vi "Kinect Example.vi"() -> ()   [LabVIEW 2011]
doc: "This example VI shows off the functionality of the new and improved Kinect API."
uses:
  Kinect Library/Kinect Type Defs/Color Image Format.ctl
  Kinect Library/Kinect Type Defs/Depth Image Format.ctl
  Kinect Library/Kinect Library.lvlib
panel:
  in  "Depth Image Format":T1
  in  "Color Image Format":T2
  in  "Kinect Sensor Index":i32
  out "Kinect Properties":T3(array[cluster])
  out "BeamAngle":dbl
  out "SoundSourceAngleConfidence":dbl
  out "SoundSourceAngle":dbl(slide) scale=-90.0..90.0
  out "Skeletal Data":T4(array[cluster])
  out "Depth Image":T5(plugin-control)
  out "Color Image":T5(plugin-control)
  in  "Stop":bool
  out "error out":errorcluster
  out "Move Success?":bool
  out "Number of Kinects Attached":i32
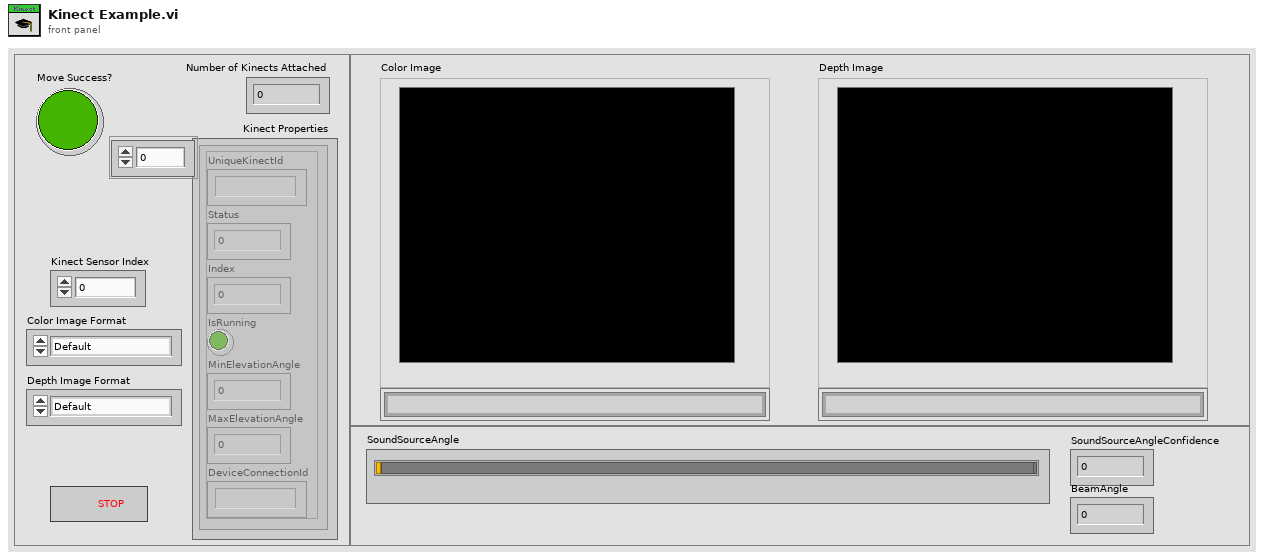
[diagram p1: front panel]
types:
  T1 = typedef "Kinect Library.lvlib/Depth Image Format.ctl" = enum16{"Default", "Undefined", "Resolution640x480Fps30", "Resolution320x240Fps30", "Resolution80x60Fps30"}
  T2 = typedef "Kinect Library.lvlib/Color Image Format.ctl" = enum16{"Default", "Undefined", "RgbResolution640x480Fps30", "RgbResolution1280x960Fps12", "YuvResolution640x480Fps15", "RawYuvResolution640x480Fps15"}
  T3 = cluster{"UniqueKinectId":string, "Status":i32, "Index":i32, "IsRunning":bool, "MinElevationAngle":i32, "MaxElevationAngle":i32, "DeviceConnectionId":string}[]
  T4 = cluster{"ClippedEdges":i32, cluster{"JointType":i32, cluster{"X":sgl, "Y":sgl, "Z":sgl}, "TrackingState":i32}[], cluster{"X":sgl, "Y":sgl, "Z":sgl}, "TrackingId":i32, "TrackingState":i32}[]
  T5 = typedef "IMAQ Image.ctl" = refnum<image>
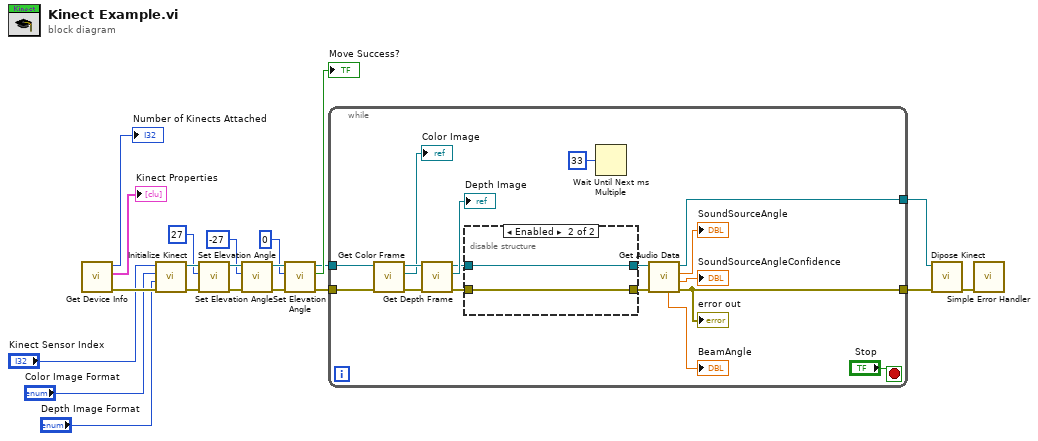
[diagram p0: block diagram]
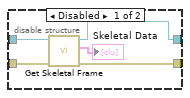
[diagram p2: hidden frame]
diagram:
  n1 = call "Get Device Info.vi"() -> ("error out"=w20:errorcluster, "Kinect Properties"=→"Kinect Properties":T3, "Number of Kinects Attached"=→"Number of Kinects Attached":i32)  [unwired: 9 in]
  n2 = call "Initialize Kinect.vi"("error in (no error)"=w20, "Depth Image Format"="Depth Image Format", "Color Image Format"="Color Image Format", "Kinect Sensor Index"="Kinect Sensor Index") -> ("error out"=w19:errorcluster, "Kinect Session out"=w15:refnum<class "Kinect Session.lvclass">)  [unwired: 6 in]
  n3 = call "Set Elevation Angle.vi"("error in (no error)"=w19, "ElevationAngle"=27, "Kinect Session in"=w15) -> ("error out"=w18:errorcluster, "Kinect Session out"=w14:refnum<class "Kinect Session.lvclass">)  [unwired: 6 in, 1 out]
  n4 = call "Set Elevation Angle.vi"("error in (no error)"=w18, "ElevationAngle"=-27, "Kinect Session in"=w14) -> ("error out"=w17:errorcluster, "Kinect Session out"=w13:refnum<class "Kinect Session.lvclass">)  [unwired: 6 in, 1 out]
  n5 = call "Set Elevation Angle.vi"("error in (no error)"=w17, "ElevationAngle"=0, "Kinect Session in"=w13) -> ("error out"=w9:errorcluster, "Success?"=→"Move Success?":bool, "Kinect Session out"=w5:refnum<class "Kinect Session.lvclass">)  [unwired: 6 in]
  n6 = while {
    tunnel: w9 -> [w37]
    tunnel: [w33] -> w8
    tunnel: w5 -> [w26]
    tunnel: [w25] -> w4
    stop <- "Stop" stop-if-true
    n7 = call "Get Color Frame.vi"("error in (no error)"=w37, "Kinect Session in"=w26) -> ("error out"=w36:errorcluster, "Color Frame"=→"Color Image":T5, "Kinect Session out"=w38:refnum<class "Kinect Session.lvclass">)  [unwired: 7 in]
    n8 = call "Get Depth Frame.vi"("error in (no error)"=w36, "Kinect Session in"=w38) -> ("error out"=w35:errorcluster, "Depth Frame"=→"Depth Image":T5, "Kinect Session out"=w24:refnum<class "Kinect Session.lvclass">)  [unwired: 7 in]
    n9 = disable-structure shown="Enabled" {
      disable-tunnel: w35 -> [w43 w45]
      disable-tunnel: [w42 w45] -> w34
      disable-tunnel: w24 -> [w40 w44]
      disable-tunnel: [w39 w44] -> w23
      frame Disabled {
        n10 = call "Get Skeletal Frame.vi"("error in (no error)"=w43, "Kinect Session in"=w40) -> ("error out"=w42:errorcluster, "Skeletal Data"=→"Skeletal Data":T4, "Kinect Session out"=w39:refnum<class "Kinect Session.lvclass">)  [unwired: 7 in]
      }
      frame Enabled {
      }
    }
    n11 = Wait Until Next ms Multiple(millisecond multiple=u32 33) -> ()  [unwired: 1 out]
    n12 = call "Get Audio Data.vi"("error in (no error)"=w34, "Kinect Session in"=w23) -> ("error out"=w33:errorcluster, "SoundSourceAngleConfidence"=→"SoundSourceAngleConfidence":dbl, "SoundSourceAngle"=→"SoundSourceAngle":dbl, "Kinect Session out"=w25:refnum<class "Kinect Session.lvclass">, "BeamAngle"=→"BeamAngle":dbl)  [unwired: 5 in]
    "error out" <- w33
  }
  n13 = call "Dipose Kinect.vi"("error in (no error)"=w8, "Kinect Session in"=w4) -> ("error out"=w7:errorcluster)  [unwired: 9 in]
  n14 = call <vilib>:"Simple Error Handler.vi"("error in (no error)"=w7) -> ()  [unwired: 4 in, 5 out]
